vi "HardwareAcquire.vi"(8 "error in (no error)":errorcluster, 11 "ESP301.lvclass":refnum<class "ESP301.lvclass">) -> (0 "error out":errorcluster, 2 "positions":dbl[](array[numeric]), 3 "ESP301.lvclass":refnum<class "ESP301.lvclass">, 4 "motor Status":T1(array[ring]), 5 "Power Status":bool[](array[boolean]))   [LabVIEW 2020, in "ESP301.lvclass"]
uses:
  ESP301.lvclass
  stop FGV control.ctl
  AcquireTypeDef.ctl
  ESP301.lvclass/ESP301.ctl
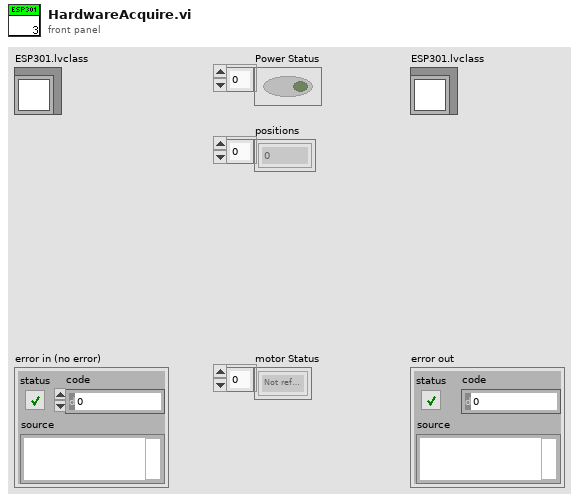
[diagram p1: front panel]
types:
  T1 = enum16{"Not referenced", "Homing", "Moving", "Ready"}[]
  T2 = typedef "AcquireTypeDef.ctl" = cluster{"busy":bool, "positions":dbl[], "Power Status":bool[], "motor Status":enum16{"Not referenced", "Homing", "Moving", "Ready"}[]}
  T3 = typedef "stop FGV control.ctl" = enum16{"Clear", "Write", "Read"}
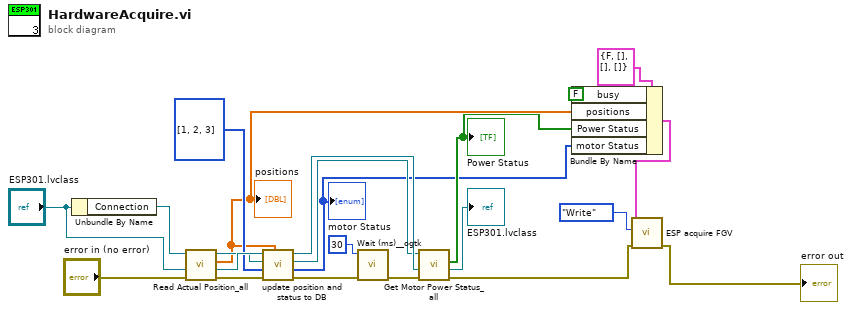
[diagram p0: block diagram]
diagram:
  n1 = Unbundle By Name("ESP301.lvclass") -> ("Connection"=w11:refnum<visa-resource-name>)
  n2 = call-dynamic "Read Actual Position_all.vi"("error in (no error)"="error in (no error)", "ESP301"="ESP301.lvclass", "VISA resource name"=w11) -> ("error out"=w10:errorcluster, "ESP301 out"=w16:refnum<class "ESP301.lvclass">, "positions"=w6:dbl[], "VISA resource name out"=w12:refnum<visa-resource-name>)  [unwired: 1 in]
  "positions" <- w6
  n3 = call "update position and status to DB.vi"("positions"=w6, "error in (no error)"=w10, "Array in"=i32[] [1, 2, 3], "VISA resource name in"=w12, "ESP301 in"=w16) -> ("error out"=w18:errorcluster, "motor Status"=w4:T1, "VISA resource name out out"=w17:refnum<visa-resource-name>, "ESP301 out"=w21:refnum<class "ESP301.lvclass">)  [unwired: 3 in]
  "motor Status" <- w4
  n4 = call "Wait (ms)__ogtk.vi"("error in (no error)"=w18, "milliseconds to wait"=u32 30) -> ("error out"=w19:errorcluster)  [unwired: 8 in, 1 out]
  n5 = call-dynamic "Get Motor Power Status_all.vi"("error in (no error)"=w19, "ESP301 in"=w21, "VISA resource name"=w17) -> ("error out"=w2:errorcluster, "ESP301 out"=→"ESP301.lvclass":refnum<class "ESP301.lvclass">, "Power Status"=w5:bool[])  [unwired: 1 in, 1 out]
  "Power Status" <- w5
  n6 = Bundle By Name(cluster=T2 {"busy"=FALSE, "positions"=[], "Power Status"=[], "motor Status"=[]} ("ESP301 Acq Data"), "busy"=FALSE, "positions"=w6, "Power Status"=w5, "motor Status"=w4) -> (w3:T2)
  n7 = call "ESP acquire FGV.vi"("error in"=w2, "Function"=stop_FGV_control."Write", "ESP301 Acq Data"=w3) -> ("error out"=→"error out":errorcluster)  [unwired: 7 in, 1 out]
